vi "GE 5565PIORC.DMA.Block.Clear (single).vi"(8 "error in (no error)":errorcluster, 10 "Block Descriptor in":T1 {"descriptor params"."data ptr (lower)" format="%.0x"; "descriptor params"."data ptr (upper)" format="%.0x"; "descriptor params"."data size" format="%.0x"; "descriptor params"."next descriptor ptr" format="%.0x"; "descriptor size" format="%08x"; "descriptor ptr (RFM)" format="%08x"; "descriptor ptr (VISA)" format="%08x"}, 11 "GE 5565PIORC in":refnum<class "GE 5565PIORC.lvclass">) -> (0 "error out":errorcluster, 2 "Block Descriptor out":T1 {"descriptor params"."data ptr (lower)" format="%.0x"; "descriptor params"."data ptr (upper)" format="%.0x"; "descriptor params"."data size" format="%.0x"; "descriptor params"."next descriptor ptr" format="%.0x"; "descriptor size" format="%08x"; "descriptor ptr (RFM)" format="%08x"; "descriptor ptr (VISA)" format="%08x"}, 3 "GE 5565PIORC out":refnum<class "GE 5565PIORC.lvclass">)   [LabVIEW 2016, in "GE 5565PIORC.lvclass"]
doc: "Sets all bytes in the provided <b>Block Descriptor</b> to zero."
uses:
  GE 5565PIORC.lvclass
  Typedefs/GE 5565PIORC.Typedef.DMA Block Descriptor.ctl
  Typedefs/GE 5565PIORC.Typedef.DMA Block Descriptor Params.ctl
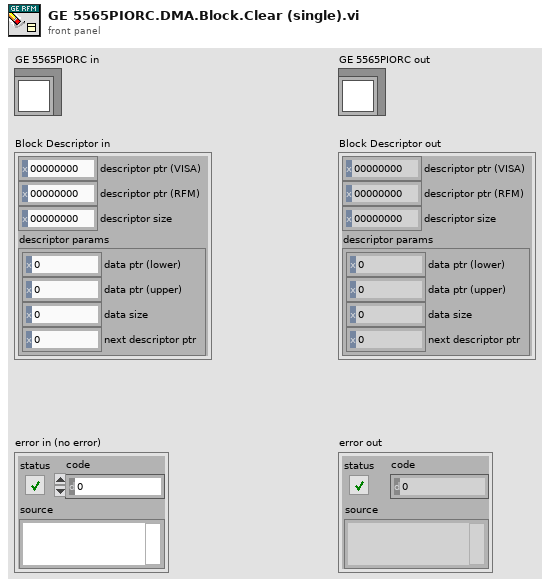
[diagram p1: front panel]
types:
  T1 = typedef "GE 5565PIORC.lvclass/GE 5565PIORC.Typedef.DMA Block Descriptor.ctl" = cluster{"descriptor ptr (VISA)":u32, "descriptor ptr (RFM)":u32, "descriptor size":u32, "descriptor params":T2}
  T2 = typedef "GE 5565PIORC.lvclass/GE 5565PIORC.Typedef.DMA Block Descriptor Params.ctl" = cluster{"data ptr (lower)":u32, "data ptr (upper)":u32, "data size":u32, "next descriptor ptr":u32}
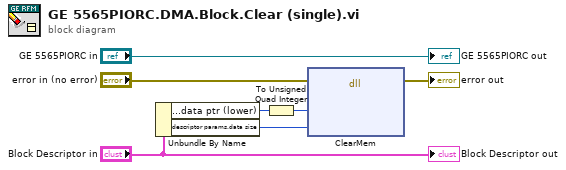
[diagram p0: block diagram]
diagram:
  n1 = Unbundle By Name("Block Descriptor in") -> ("descriptor params.data ptr (lower)"=w3:u32, "descriptor params.data size"=w2:u32)
  n2 = To Unsigned Quad Integer(1:w3) -> (0:w1:u64)
  n3 = dll-call lib="LabVIEW" fn="ClearMem"(error in="error in (no error)", "pointer"=w1, "size"=w2) -> (error out=→"error out":errorcluster)  [unwired: 5 in, 1 out]
  "GE 5565PIORC out" <- "GE 5565PIORC in"
  "Block Descriptor out" <- "Block Descriptor in"
